vi "SRV_Check File Exists with Dialog.vi"(0 "Filepath":path, 1 "File Type":string="Motor Config File", 11 "error in (no error)":errorcluster) -> (4 "Filepath dup":path, 10 "File Exists?":bool, 15 "error out":errorcluster)   [LabVIEW 2009]
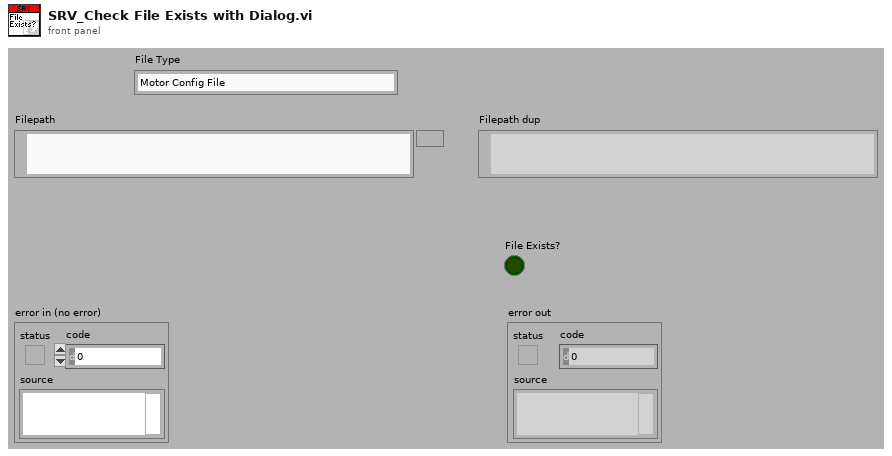
[diagram p1: front panel]
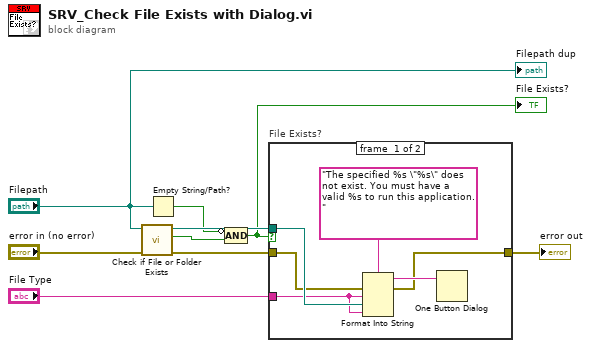
[diagram p0: block diagram]
diagram:
  n1 = call <vilib>:"Check if File or Folder Exists.vi"("error in (no error)"="error in (no error)", "path"="Filepath") -> ("error out"=w8:errorcluster, "file or folder exists?"=w2:bool, "dup path"=w7:path)  [unwired: 7 in]
  n2 = Empty String/Path?(string/path="Filepath") -> (empty?=w3:bool)
  n3 = Compound Arithmetic op=AND(invert w3, w2) -> (w1:bool)
  "File Exists?" <- w1
  n4 = case "File Exists?" shown="False" w1 {
    tunnel: w8 -> [w11 w16]
    tunnel: w7 -> [w15 _]
    tunnel: "File Type" -> [w14 _]
    tunnel: [w10 w16] -> w5
    frame #0 {
      n5 = Format Into String(format string="The specified %s \"%s\" does not exist. You must have a valid %s to run this application.", error in=w11, w14, w15, w14) -> (resulting string=w12:string, error out=w10:errorcluster)  [unwired: 1 in]
      n6 = One Button Dialog(message=w12) -> ()  [unwired: 1 in, 1 out]
    }
    frame #1 {
    }
  }
  "error out" <- w5
  "Filepath dup" <- "Filepath"
